vi "XYZ.vi"(0 "Function":T9, 2 "Notifications":T3, 3 "Refnums":T4, 5 "Connection Settings":T5={"Tango VISA"="", "Baudrate"=57600, "Show Protocol?"=FALSE}, 7 "Coordinate Control":T1, 9 "Manual Control":T6 {"Z step" scale=0.1..10.0; "XY Step" scale=0.1..1000.0}, 11 "Error In (no error)":errorcluster) -> (6 "Status":T8, 8 "LimitsOutput":T7[](array[typedef]), 15 "Error Out":errorcluster caption="Error out")   [LabVIEW 2014]
uses:
  XYZ Function.ctl
  <instrlib>/Tango Drivers/Labview/SubVIs/Axis_Switch.ctl
  XYZ Stage Control.ctl
  XYZ Connection Settings.ctl
  XYZ Refnums.ctl
  support/Instrument Status.ctl
  XYZ Notifications.ctl
  XYZ Coordinate Control.ctl
  support/Instrument Status State.ctl
  <userlib>/Tango_DLL/Tango_DLL.lvlib
panel:
  out "Instrument Status":T2
  out "Range Measurement":cluster{"Measured?":bool, "Range":dbl[]}={"Measured?"=TRUE, "Range"=[]}
  # "LICENSED MATERIALS – PROPERTY OF IBM\nCopyright IBM Corp. 2016,\nALL RIGHTS RESERVED"
  # "XY"
  # "Z"
  # "XY"
  # "Z"
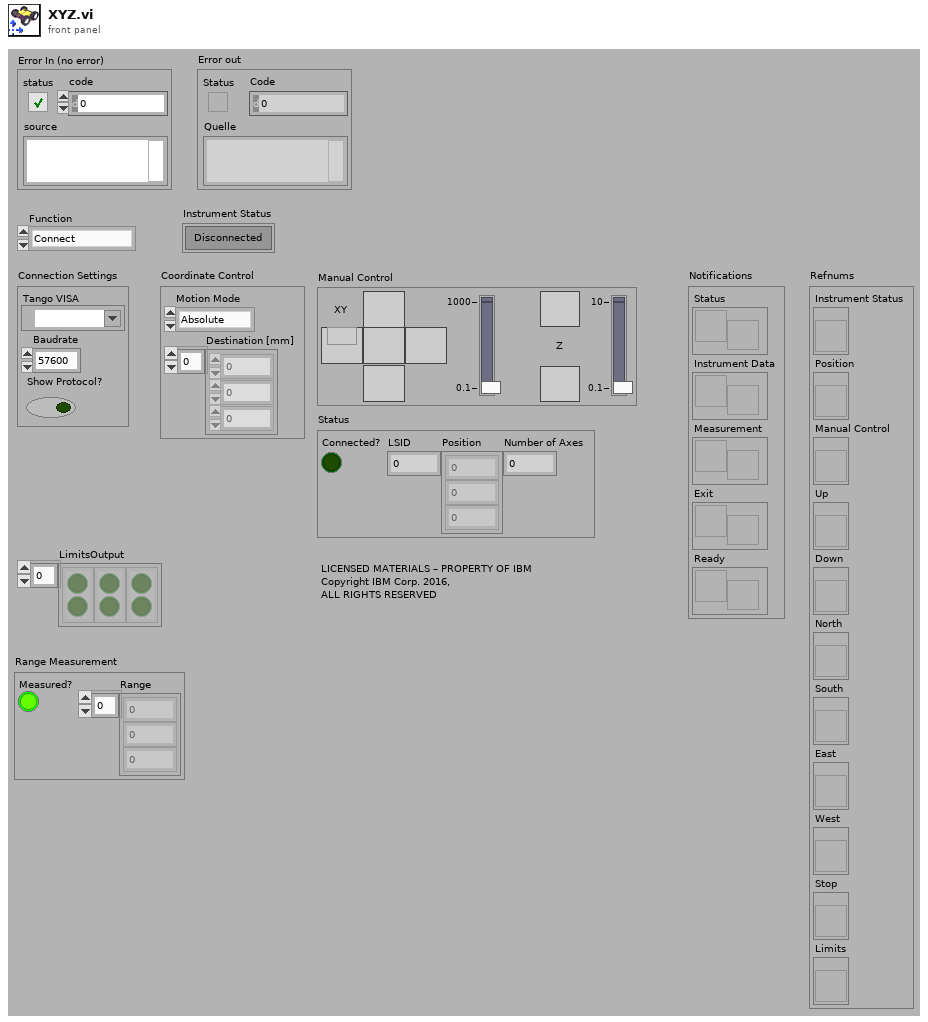
[diagram p1: front panel]
types:
  T1 = typedef "XYZ Coordinate Control.ctl" = cluster{"Motion Mode":enum16{"Absolute", "Relative"}, "Destination [mm]":dbl[]}
  T2 = typedef "Instrument Status.ctl" = bool
  T3 = typedef "XYZ Notifications.ctl" = cluster{"Status":refnum<notifier>, "Instrument Data":refnum<notifier>, "Measurement":refnum<notifier>, "Exit":refnum<notifier>, "Ready":refnum<notifier>}
  T4 = typedef "XYZ Refnums.ctl" = cluster{"Instrument Status":refnum<vi>, "Position":refnum<vi>, "Manual Control":refnum<vi>, "Up":refnum<vi>, "Down":refnum<vi>, "North":refnum<vi>, "South":refnum<vi>, "East":refnum<vi>, "West":refnum<vi>, "Stop":refnum<vi>, "Limits":refnum<vi>}
  T5 = typedef "XYZ Connection Settings.ctl" = cluster{"Tango VISA":refnum<visa-resource-name>, "Baudrate":i32, "Show Protocol?":bool}
  T6 = typedef "XYZ Stage Control.ctl" = cluster{"North":bool, "South":bool, "West":bool, "East":bool, "Up":bool, "Down":bool, "Stop":bool, "XY Step":dbl, "Z step":dbl}
  T7 = typedef "Axis_Switch.ctl" = cluster{"E0":bool, "EE":bool}
  T8 = cluster{"Connected?":bool, "LSID":i32, "Position":dbl[], "Number of Axes":u8}
  T9 = typedef "XYZ Function.ctl" = enum16{"Connect", "Initialize", "Calibrate", "Meaure Range", "Limits", "Center", "Set Zero", "Velocity", "Manual Control", "Coordinate Move", "Move with Backlash Compensation", "Meander", "Sequence", "Analog Output", "Send Command", "Show Protocol", "Get Status", "Disconnect", "Update Refnums"}
  T10 = typedef "Instrument Status State.ctl" = enum16{"Unknown", "Idle", "Standby", "Configuring", "Measuring", "Moving", "Disconnected"}
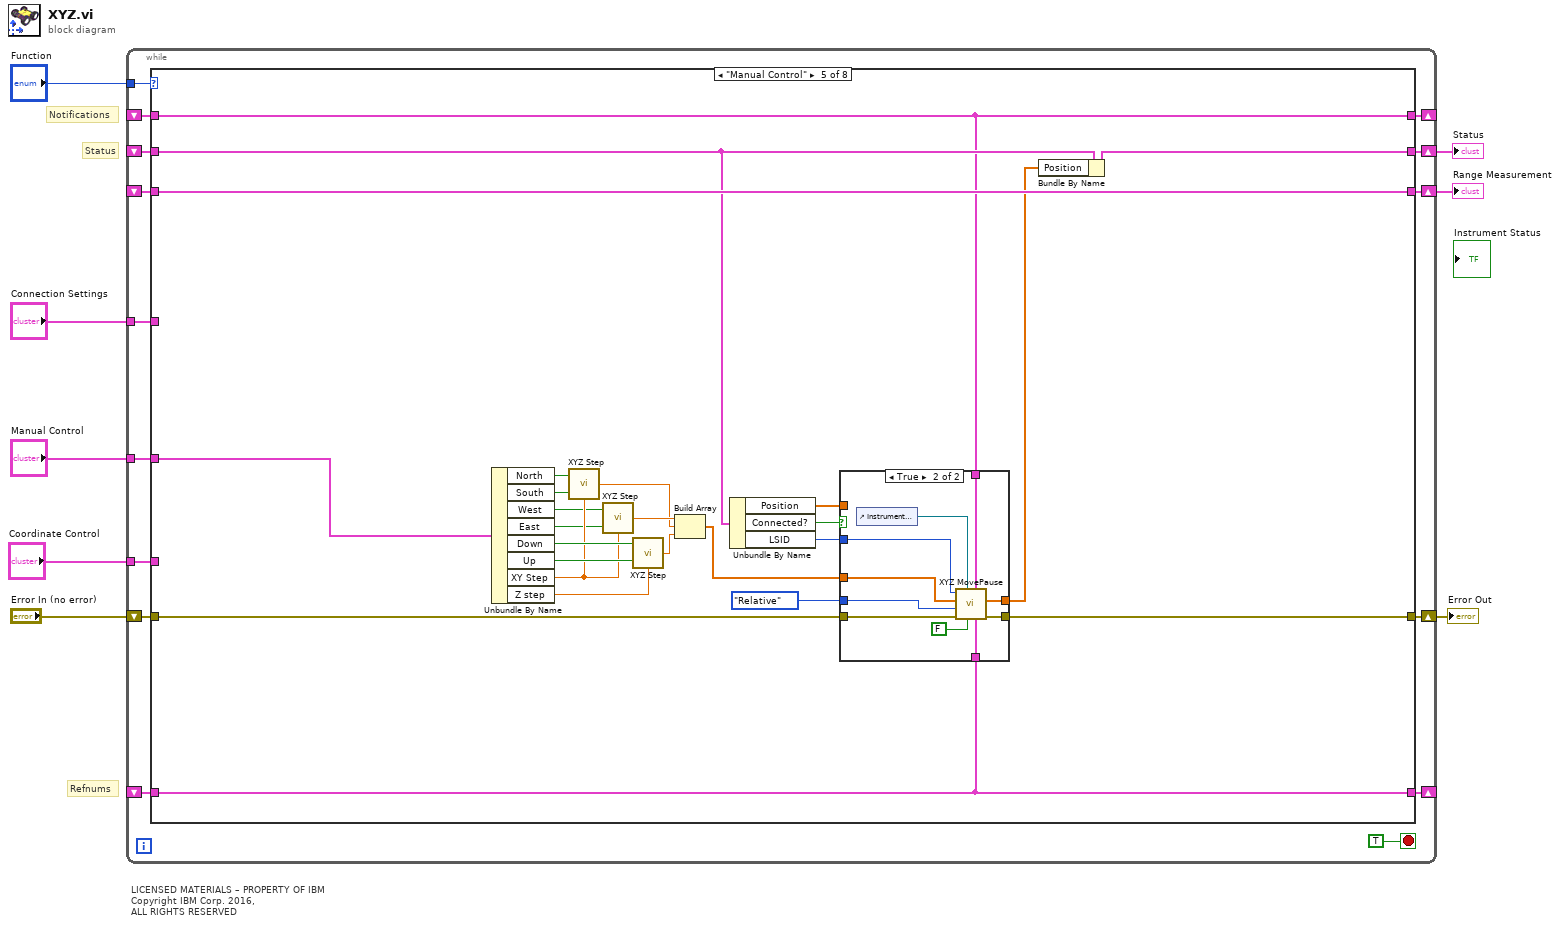
[diagram p0: block diagram]
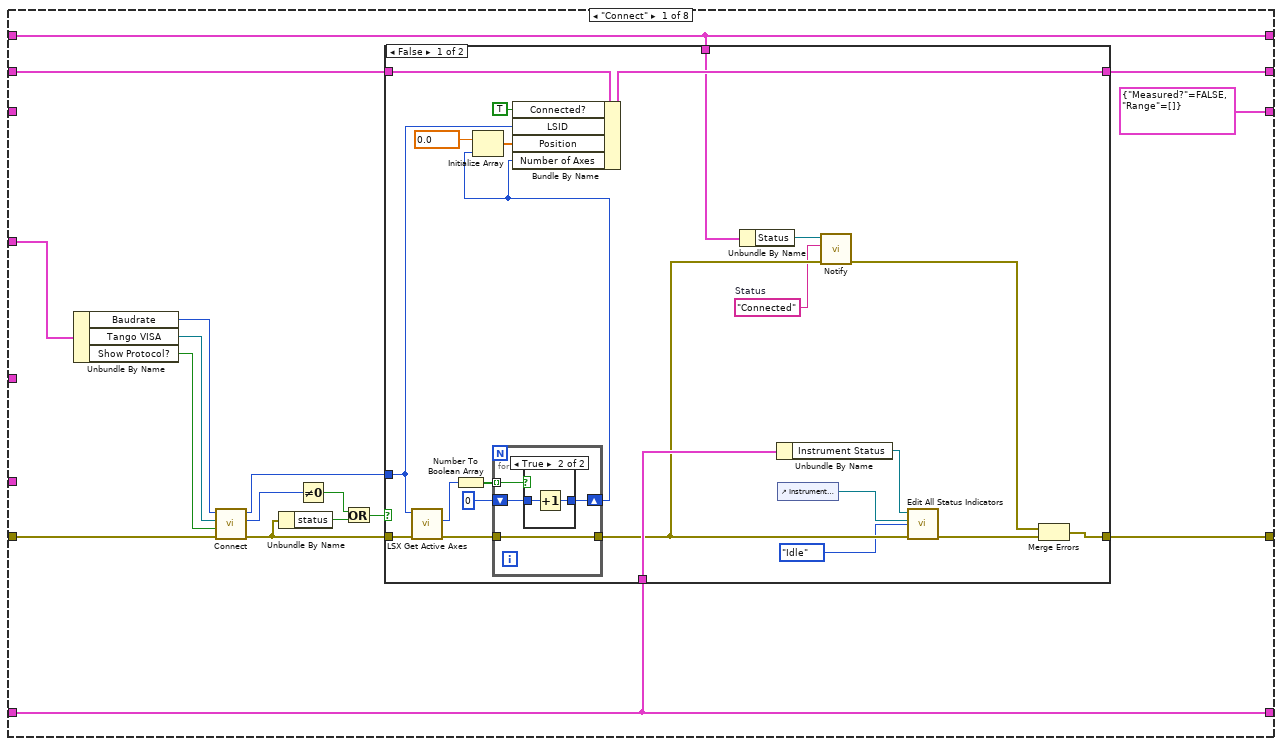
[diagram p2: hidden frame]
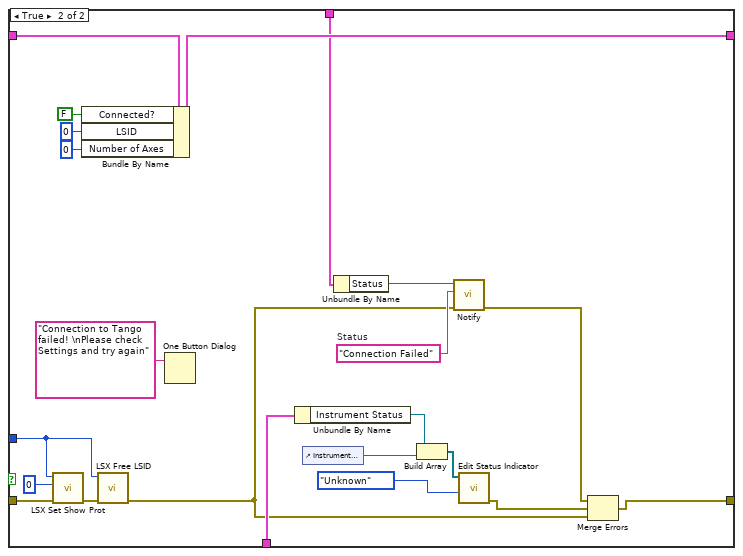
[diagram p4: hidden frame]
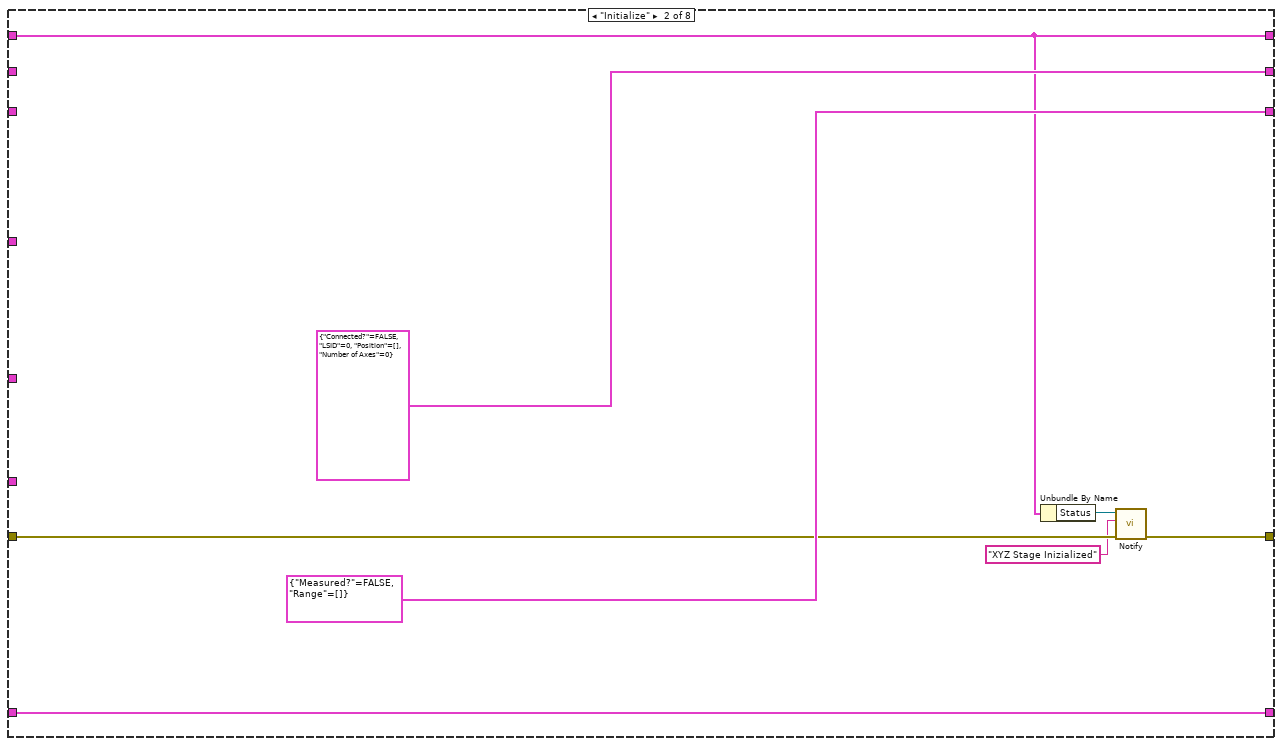
[diagram p5: hidden frame]
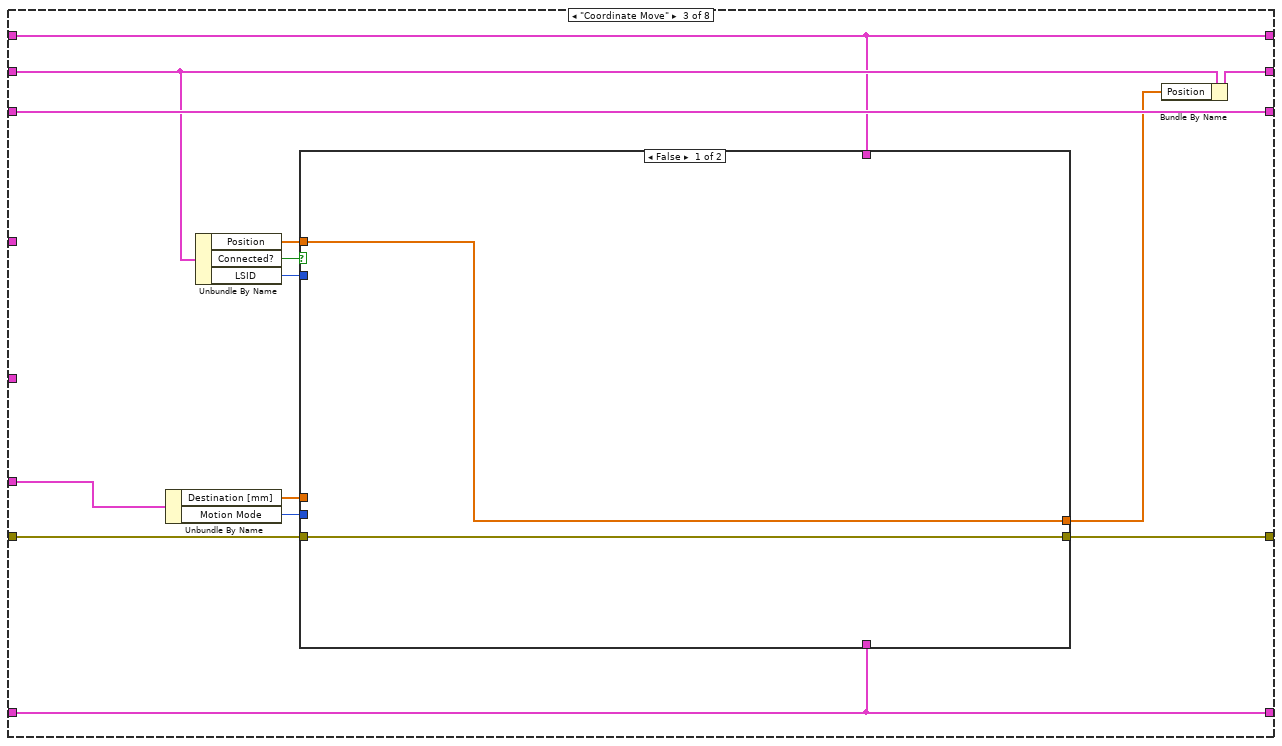
[diagram p6: hidden frame]
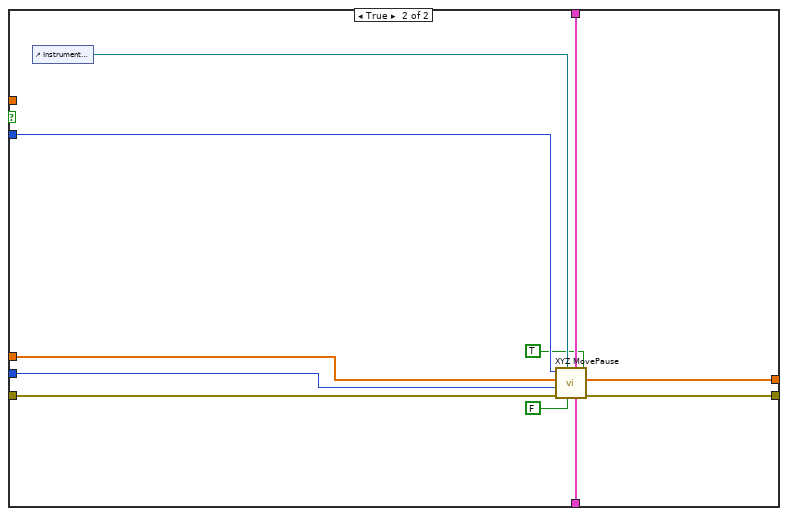
[diagram p7: hidden frame]
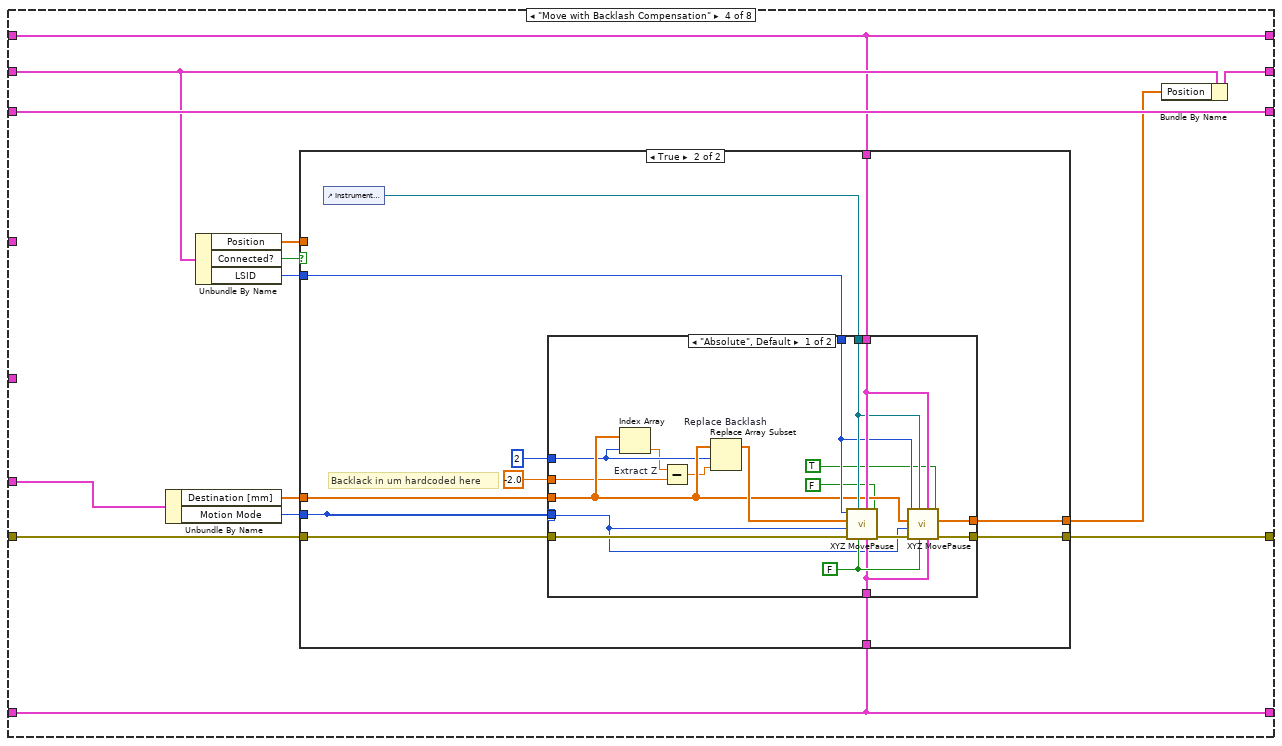
[diagram p8: hidden frame]
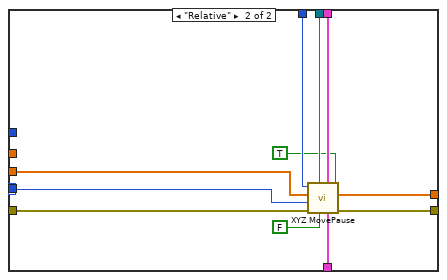
[diagram p10: hidden frame]
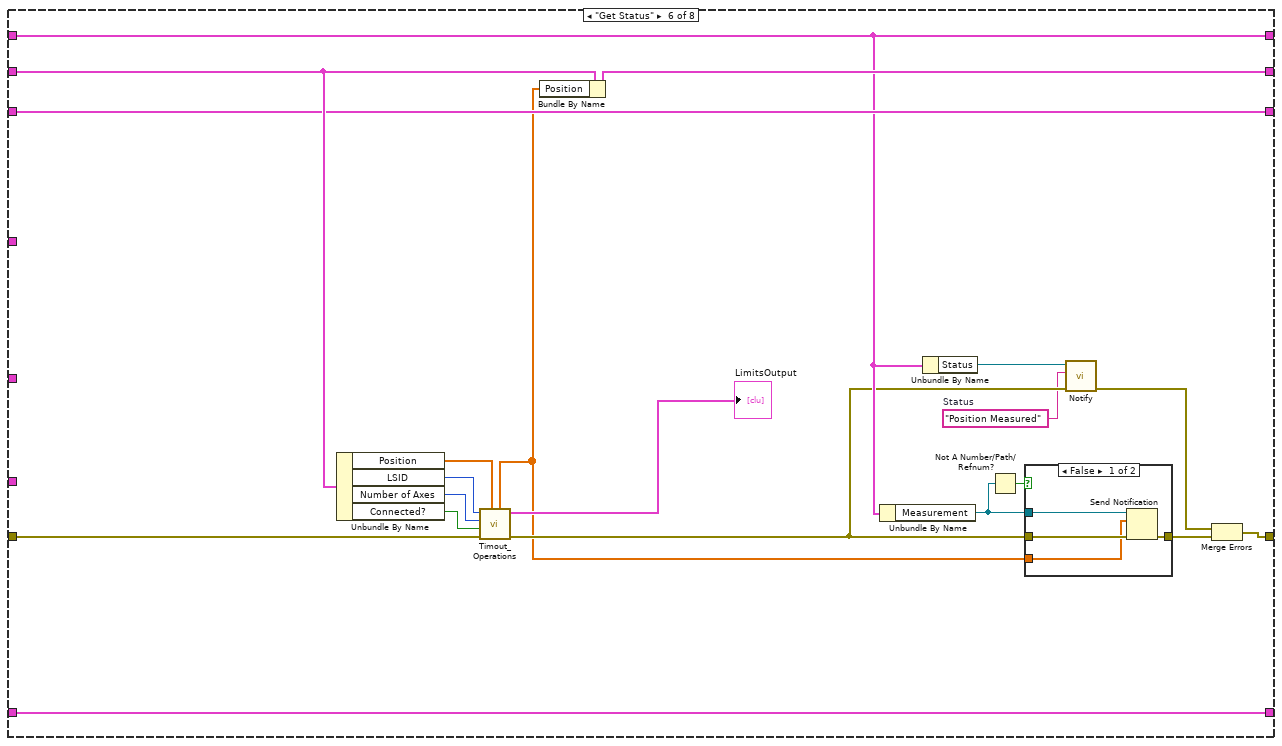
[diagram p12: hidden frame]
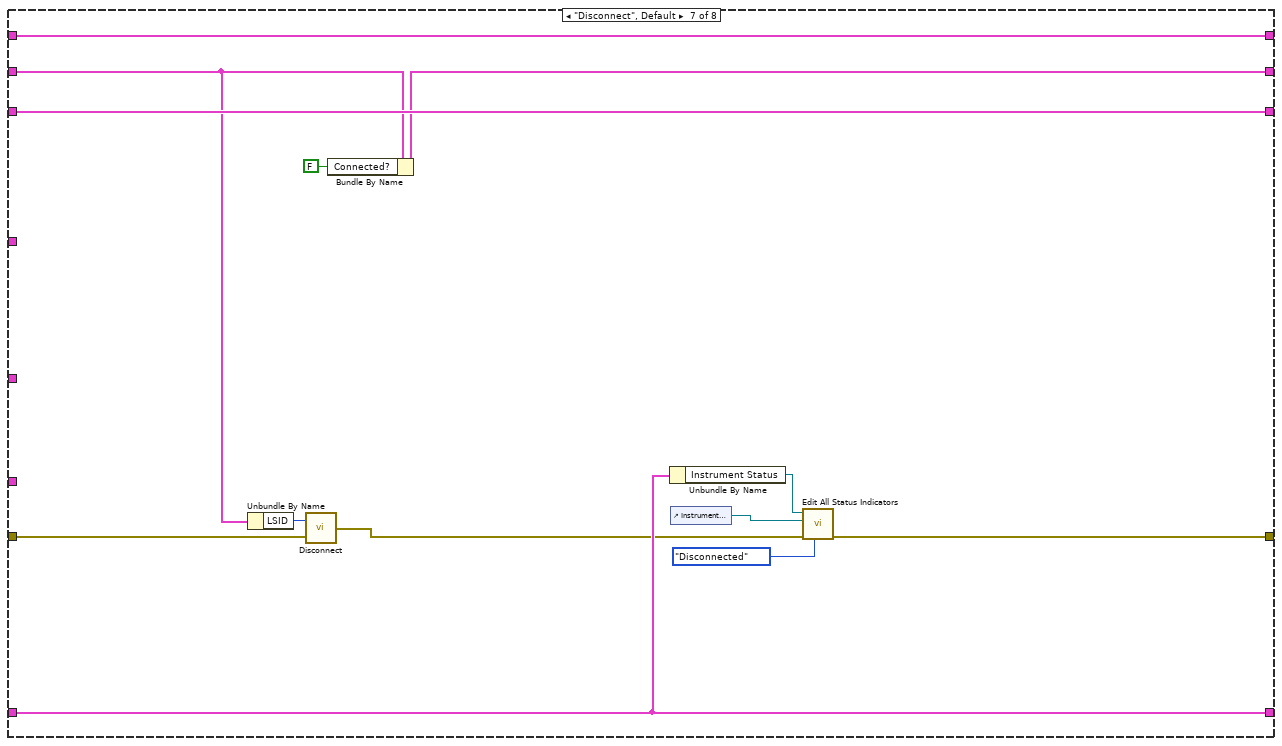
[diagram p14: hidden frame]
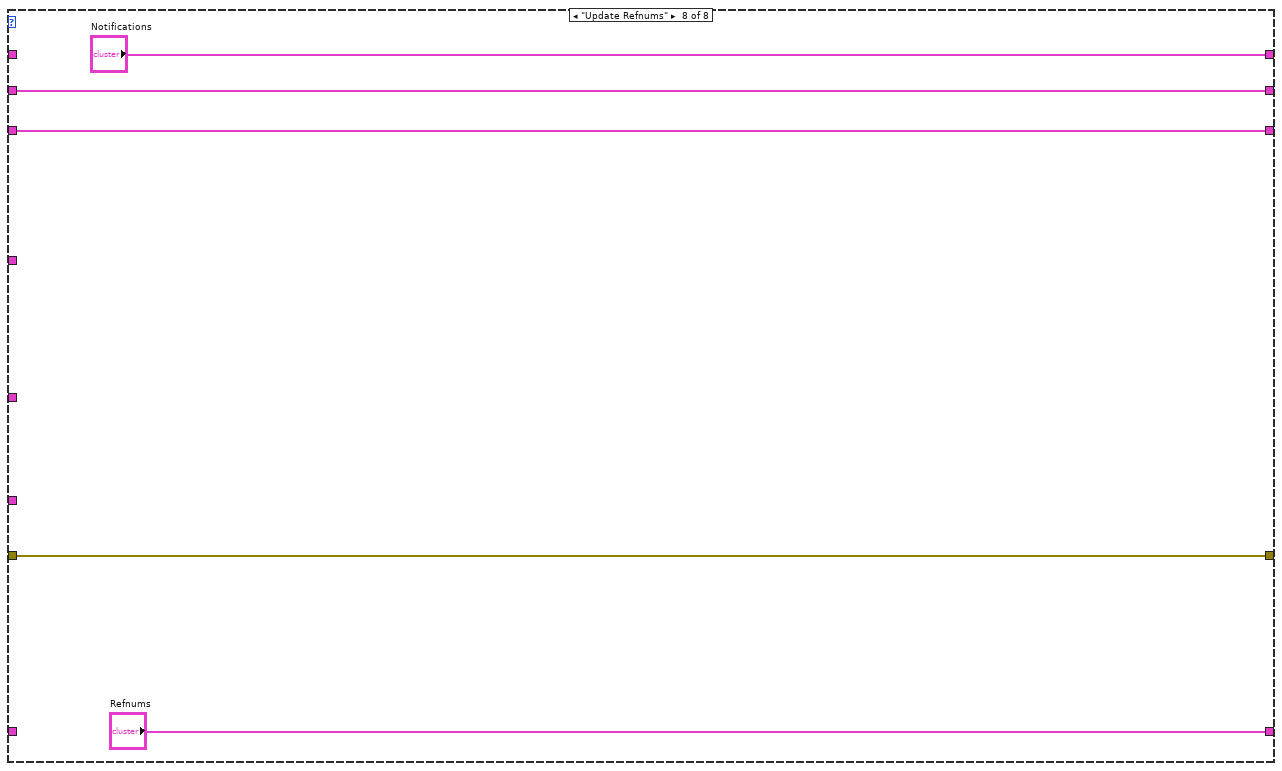
[diagram p15: hidden frame]
diagram:
  # "LICENSED MATERIALS – PROPERTY OF IBM\nCopyright IBM Corp. 2016,\nALL RIGHTS RESERVED"
  # "Status"
  # "Refnums"
  # "Notifications"
  n1 = while {
    tunnel: "Function" -> [w23]
    shift-right: [w22] -> w7
    shift-left: _ -> [w21]
    shift-right: [w19] -> w5
    shift-left: "Error In (no error)" -> [w20]
    shift-right: [w18] -> w4
    shift-left: _ -> [w17]
    tunnel: "Connection Settings" -> [w15]
    shift-right: [w14] -> _
    shift-left: _ -> [w13]
    shift-right: [w12] -> _
    shift-left: _ -> [w11]
    tunnel: "Coordinate Control" -> [w10]
    tunnel: "Manual Control" -> [w9]
    stop <- TRUE stop-if-true
    n2 = case shown="\"Manual Control\"" w23 {
      tunnel: [w31 T8 {"Connected?"=FALSE, "LSID"=0, "Position"=[], "Number of Axes"=0} ("Status 2") w108 w135 w190 w234 w254 w260] -> w22
      tunnel: w21 -> [w32 _ w109 w136 w189 w238 w255 w260]
      tunnel: w20 -> [w40 w95 w113 w140 w207 w240 w257 w263]
      tunnel: [w35 w93 w104 w131 w186 w225 w249 w263] -> w19
      tunnel: [cluster{"Measured?":bool, "Range":dbl[]} {"Measured?"=FALSE, "Range"=[]} ("Range Measurement 3") cluster{"Measured?":bool, "Range":dbl[]} {"Measured?"=FALSE, "Range"=[]} ("Range Measurement 3") w114 w141 w208 w232 w256 w259] -> w18
      tunnel: w17 -> [_ _ w114 w141 w208 w232 w256 w259]
      tunnel: w15 -> [w29 _ _ _ _ _ _ _]
      tunnel: [w24 w96 w105 w132 w188 w227 w252 "Notifications"] -> w14
      tunnel: w13 -> [w24 w96 w105 w132 w188 w227 w252 _]
      tunnel: [w25 w98 w111 w138 w204 w231 w251 "Refnums"] -> w12
      tunnel: w11 -> [w25 w98 w111 w138 w204 w231 w251 _]
      tunnel: w10 -> [_ _ w101 w128 _ _ _ _]
      tunnel: w9 -> [_ _ _ _ w184 _ _ _]
      frame "Connect" {
        n3 = Unbundle By Name(w29) -> ("Baudrate"=w28:i32, "Tango VISA"=w26:refnum<visa-resource-name>, "Show Protocol?"=w27:bool)
        n4 = call <instrlib>:"Connect.vi"("error in (no error)"=w40, "ShProt?"=w27, "pcAComName"=w26, "lABaudRate"=w28) -> ("error out"=w36:errorcluster, "function return"=w37:i32, "plLSID out"=w34:i32)  [unwired: 4 in]
        n5 = Unbundle By Name(w36) -> ("status"=w39:bool)
        n6 = Not Equal To 0?(x=w37) -> (x != 0?=w38:bool)
        n7 = Or(x=w38, y=w39) -> (x .or. y?=w33:bool)
        n8 = case shown="False" w33 {
          tunnel: w36 -> [w63 w90]
          tunnel: [w46 w81] -> w35
          tunnel: w34 -> [w55 w89]
          tunnel: w32 -> [w62 w87]
          tunnel: [w61 w86] -> w31
          tunnel: w25 -> [w50 w82]
          tunnel: w24 -> [w48 w75]
          frame False {
            w45 = "Connected"  # Status
            n9 = call <userlib>:"LSX Get Active Axes.vi"("error in (no error)"=w63, "lLSID"=w55) -> ("error out"=w58:errorcluster, "plFlags out"=w57:i32)  [unwired: 7 in, 1 out]
            n10 = Number To Boolean Array(number=w57) -> (Boolean array=w56:bool[])
            n11 = for {
              tunnel: w56 -> [w67] mode=indexing
              shift-right: [w65] -> w54
              shift-left: u8 0 -> [w66]
              tunnel: [w64] -> w47
              tunnel: w58 -> [w64]
              n12 = case shown="True" w67 {
                tunnel: w66 -> [w68 w70]
                tunnel: [w68 w69] -> w65
                frame False {
                }
                frame True {
                  n13 = Increment(x=w70) -> (x+1=w69:u8)
                }
              }
            }
            n14 = Initialize Array(0.0, w54) -> (w52:dbl[])
            n15 = Bundle By Name(cluster=w62, "Connected?"=TRUE, "LSID"=w55, "Position"=w52, "Number of Axes"=w54) -> (w61:T8)
            n16 = Unbundle By Name(w48) -> ("Status"=w49:refnum<notifier>)
            n17 = Unbundle By Name(w50) -> ("Instrument Status"=w43:refnum<vi>)
            n18 = control-ref of="Instrument Status"() -> (w42:refnum<vi>)
            n19 = call "Notify.vi"("error in (no error)"=w47, "String"=w45, "Notifier in"=w49) -> ("error out"=w44:errorcluster)  [unwired: 8 in]
            n20 = call "Edit All Status Indicators.vi"("Instrument Status Ouside"=w43, "Instrument Status Inside"=w42, "Error In"=w47, "State"=Instrument_Status_State."Idle") -> ("Error Out"=w51:errorcluster)  [unwired: 6 in]
            n21 = Merge Errors(w44, w51) -> (w46:errorcluster)
          }
          frame True {
            w73 = "Connection Failed"  # Status
            n22 = call <userlib>:"LSX Set Show Prot.vi"("error in (no error)"=w90, "bShowProt"=0, "lLSID"=w89) -> ("error out"=w91:errorcluster)  [unwired: 7 in, 1 out]
            n23 = Bundle By Name(cluster=w87, "Connected?"=FALSE, "LSID"=0, "Number of Axes"=u8 0) -> (w86:T8)
            n24 = call <userlib>:"LSX Free LSID.vi"("error in (no error)"=w91, "lLSID"=w89) -> ("error out"=w72:errorcluster)  [unwired: 8 in, 1 out]
            n25 = One Button Dialog(message="Connection to Tango failed! \nPlease check Settings and try again" ("Nachricht")) -> ()  [unwired: 1 in, 1 out]
            n26 = Unbundle By Name(w82) -> ("Instrument Status"=w76:refnum<vi>)
            n27 = control-ref of="Instrument Status"() -> (w79:refnum<vi>)
            n28 = Unbundle By Name(w75) -> ("Status"=w74:refnum<notifier>)
            n29 = Build Array(w76, w79) -> (w78:refnum<vi>[])
            n30 = call "Notify.vi"("error in (no error)"=w72, "String"=w73, "Notifier in"=w74) -> ("error out"=w71:errorcluster)  [unwired: 8 in]
            n31 = call "Edit Status Indicator.vi"("State"=Instrument_Status_State."Unknown", "Instrument Status Refnum"=w78) -> ("error out"=w77:errorcluster)  [unwired: 2 in, 7 out]
            n32 = Merge Errors(w71, w77, w72) -> (w81:errorcluster)
          }
        }
      }
      frame "Initialize" {
        n33 = Unbundle By Name(w96) -> ("Status"=w97:refnum<notifier>)
        n34 = call "Notify.vi"("error in (no error)"=w95, "String"="XYZ Stage Inizialized", "Notifier in"=w97) -> ("error out"=w93:errorcluster)  [unwired: 8 in]
      }
      frame "Coordinate Move" {
        n35 = Unbundle By Name(w101) -> ("Destination [mm]"=w106:dbl[], "Motion Mode"=w107:enum16{"Absolute", "Relative"})
        n36 = Unbundle By Name(w109) -> ("Position"=w103:dbl[], "Connected?"=w110:bool, "LSID"=w112:i32)
        n37 = case shown="False" w110 {
          tunnel: w105 -> [_ w127]
          tunnel: w113 -> [w116 w126]
          tunnel: [w116 w125] -> w104
          tunnel: w112 -> [_ w124]
          tunnel: w106 -> [_ w120]
          tunnel: w107 -> [_ w119]
          tunnel: w111 -> [_ w123]
          tunnel: w103 -> [w115 _]
          tunnel: [w115 w121] -> w102
          frame False {
          }
          frame True {
            n38 = control-ref of="Instrument Status"() -> (w122:refnum<vi>)
            n39 = call "XYZ MovePause.vi"("Notify?"=TRUE, "Refnums"=w123, "Notifications"=w127, "Wait For Motion Done?"=FALSE, "Instrument Status"=w122, "error in (no error)"=w126, "Motion Mode"=w119, "Destination [mm]"=w120, "LSID"=w124) -> ("error out"=w125:errorcluster, "Position"=w121:dbl[])  [unwired: 1 in]
          }
        }
        n40 = Bundle By Name(cluster=w109, "Position"=w102) -> (w108:T8)
      }
      frame "Move with Backlash Compensation" {
        n41 = Unbundle By Name(w128) -> ("Destination [mm]"=w133:dbl[], "Motion Mode"=w134:enum16{"Absolute", "Relative"})
        n42 = Unbundle By Name(w136) -> ("Position"=w130:dbl[], "Connected?"=w137:bool, "LSID"=w139:i32)
        n43 = case shown="True" w137 {
          tunnel: w132 -> [_ w154]
          tunnel: w140 -> [w143 w153]
          tunnel: [w143 w152] -> w131
          tunnel: w139 -> [_ w151]
          tunnel: w133 -> [_ w147]
          tunnel: w134 -> [_ w146]
          tunnel: w138 -> [_ w150]
          tunnel: w130 -> [w142 _]
          tunnel: [w142 w148] -> w129
          frame False {
          }
          frame True {
            # "Backlack in um hardcoded here"
            n44 = control-ref of="Instrument Status"() -> (w149:refnum<vi>)
            n45 = case shown="\"Absolute\", Default" w146 {
              selector: w146 -> [w155 w182]
              tunnel: w153 -> [w172 w181]
              tunnel: w146 -> [_ _]
              tunnel: w154 -> [w170 w178]
              tunnel: w149 -> [w169 w179]
              tunnel: w151 -> [w168 w180]
              tunnel: w150 -> [w166 w177]
              tunnel: [w165 w173] -> w148
              tunnel: [w164 w176] -> w152
              tunnel: w147 -> [w162 w174]
              tunnel: 2 ("index") -> [w161 _]
              tunnel: -2.0 ("y") -> [w158 _]
              frame "Absolute", Default {
                w167 = FALSE ("Wait For Motion Done?")
                n46 = Index Array "Extract Z"(array=w162, index=w161) -> (element=w159:dbl)
                n47 = Subtract(x=w159, y=w158) -> (x-y=w160:dbl)
                n48 = Replace Array Subset "Replace Backlash"(array=w162, new element=w160, index=w161) -> (w163:dbl[])
                n49 = call "XYZ MovePause.vi"("Notify?"=FALSE, "Refnums"=w166, "Notifications"=w170, "Wait For Motion Done?"=w167, "Instrument Status"=w169, "error in (no error)"=w172, "Motion Mode"=w155, "Destination [mm]"=w163, "LSID"=w168) -> ("error out"=w171:errorcluster)  [unwired: 1 in, 1 out]
                n50 = call "XYZ MovePause.vi"("Notify?"=TRUE, "Refnums"=w166, "Notifications"=w170, "Wait For Motion Done?"=w167, "Instrument Status"=w169, "error in (no error)"=w171, "Motion Mode"=w155, "Destination [mm]"=w162, "LSID"=w168) -> ("error out"=w164:errorcluster, "Position"=w165:dbl[])  [unwired: 1 in]
              }
              frame "Relative" {
                n51 = call "XYZ MovePause.vi"("Notify?"=TRUE, "Refnums"=w177, "Notifications"=w178, "Wait For Motion Done?"=FALSE, "Instrument Status"=w179, "error in (no error)"=w181, "Motion Mode"=w182, "Destination [mm]"=w174, "LSID"=w180) -> ("error out"=w176:errorcluster, "Position"=w173:dbl[])  [unwired: 1 in]
              }
            }
          }
        }
        n52 = Bundle By Name(cluster=w136, "Position"=w129) -> (w135:T8)
      }
      frame "Manual Control" {
        n53 = Unbundle By Name(w184) -> ("North"=w202:bool, "South"=w201:bool, "West"=w196:bool, "East"=w195:bool, "Down"=w200:bool, "Up"=w199:bool, "XY Step"=w198:dbl, "Z step"=w197:dbl)
        n54 = call "XYZ Step.vi"("Step Size"=w198, "Negative"=w201, "Positive"=w202) -> ("Relative Movement"=w193:dbl)
        n55 = call "XYZ Step.vi"("Step Size"=w198, "Negative"=w195, "Positive"=w196) -> ("Relative Movement"=w194:dbl)
        n56 = call "XYZ Step.vi"("Step Size"=w197, "Negative"=w199, "Positive"=w200) -> ("Relative Movement"=w192:dbl)
        n57 = Build Array(w194, w193, w192) -> (w191:dbl[])
        n58 = Unbundle By Name(w189) -> ("Position"=w185:dbl[], "Connected?"=w203:bool, "LSID"=w206:i32)
        n59 = case shown="True" w203 {
          tunnel: w188 -> [_ w220]
          tunnel: w207 -> [w210 w219]
          tunnel: [w210 w218] -> w186
          tunnel: w206 -> [_ w217]
          tunnel: w191 -> [_ w216]
          tunnel: enum16{"Absolute", "Relative"}."Relative" ("Motion Mode") -> [_ w215]
          tunnel: w204 -> [_ w213]
          tunnel: [w209 w211] -> w187
          tunnel: w185 -> [w209 _]
          frame False {
          }
          frame True {
            n60 = control-ref of="Instrument Status"() -> (w212:refnum<vi>)
            n61 = call "XYZ MovePause.vi"("Refnums"=w213, "Notifications"=w220, "Wait For Motion Done?"=FALSE, "Instrument Status"=w212, "error in (no error)"=w219, "Motion Mode"=w215, "Destination [mm]"=w216, "LSID"=w217) -> ("error out"=w218:errorcluster, "Position"=w211:dbl[])  [unwired: 2 in]
          }
        }
        n62 = Bundle By Name(cluster=w189, "Position"=w187) -> (w190:T8)
      }
      frame "Get Status" {
        w221 = "Position Measured"  # Status
        n63 = Unbundle By Name(w238) -> ("Position"=w235:dbl[], "LSID"=w239:i32, "Number of Axes"=w237:u8, "Connected?"=w236:bool)
        n64 = call <instrlib>:"Timout_Operations.vi"("PosIn"=w235, "error in"=w240, "Connected?"=w236, "NumberOfAxes"=w237, "plLSID"=w239) -> ("error out"=w226:errorcluster, "LimitsOutput"=→"LimitsOutput":T7[], "PosOut"=w222:dbl[])  [unwired: 2 in, 2 out]
        n65 = Bundle By Name(cluster=w238, "Position"=w222) -> (w234:T8)
        n66 = Unbundle By Name(w227) -> ("Measurement"=w230:refnum<notifier>)
        n67 = Unbundle By Name(w227) -> ("Status"=w228:refnum<notifier>)
        n68 = Not A Number/Path/Refnum?(number/path/refnum=w230) -> (NaN/Path/Refnum?=w229:bool)
        n69 = case shown="False" w229 {
          tunnel: w230 -> [w244 _]
          tunnel: w226 -> [w243 w245]
          tunnel: [w242 w245] -> w223
          tunnel: w222 -> [w241 _]
          frame False {
            n70 = Send Notification(notification=w241, notifier=w244, error in (no error)=w243) -> (error out=w242:errorcluster)  [unwired: 1 out]
          }
          frame True {
          }
        }
        n71 = call "Notify.vi"("error in (no error)"=w226, "String"=w221, "Notifier in"=w228) -> ("error out"=w224:errorcluster)  [unwired: 8 in]
        n72 = Merge Errors(w224, w223) -> (w225:errorcluster)
      }
      frame "Disconnect", Default {
        n73 = Unbundle By Name(w255) -> ("LSID"=w258:i32)
        n74 = call <instrlib>:"Disconnect.vi"("error in (no error)"=w257, "lLSID"=w258) -> ("error out"=w250:errorcluster)
        n75 = Bundle By Name(cluster=w255, "Connected?"=FALSE) -> (w254:T8)
        n76 = Unbundle By Name(w251) -> ("Instrument Status"=w248:refnum<vi>)
        n77 = control-ref of="Instrument Status"() -> (w247:refnum<vi>)
        n78 = call "Edit All Status Indicators.vi"("Instrument Status Ouside"=w248, "Instrument Status Inside"=w247, "Error In"=w250, "State"=Instrument_Status_State."Disconnected") -> ("Error Out"=w249:errorcluster)  [unwired: 6 in]
      }
      frame "Update Refnums" {
      }
    }
  }
  "Status" <- w7
  "Error Out" <- w5
  "Range Measurement" <- w4
